vi "Parse WebMessage JSON.vi"(11 "JSON in":string) -> (2 "Data out":string, 3 "Type out":string)   [LabVIEW 2020, in "WebView.lvclass"]
uses:
  WebView_class/WebView.lvclass
  <vilib>/JDP Science/JSONtext/LVClass Serializer/JSONtext LVClass Serializer.lvclass
  <vilib>/JDP Science/JSONtext/JSONtext.lvlib
  578b13ae-8167-4477-89af-624874bd8b4a.vi
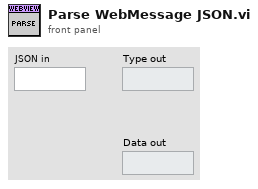
[diagram p1: front panel]
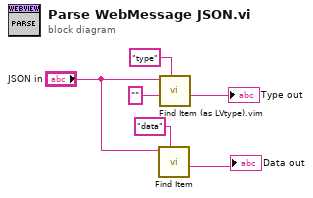
[diagram p0: block diagram]
diagram:
  n1 = call <vilib>:"Find Item.vi"("$Path or Item Name"="data", "JSON"="JSON in") -> ("<JSON>"=→"Data out":string)  [unwired: 6 in, 3 out]
  n2 = call "Find Item (as LVtype).vim"("$Path or Item Name"="type", "Data Type and Default Value"="", "JSON"="JSON in") -> ("Data"=→"Type out":string)  [unwired: 5 in, 3 out]
